vi "ODMR_MW_pulses_0.5pi(1,2,3).vi"(7 "pi/2 duration [ns]":i64=100, 9 "Measurement time [ns]":i64=100, 10 "tau/2 duration [ns]":u32, 11 "PulsePattern in":refnum<class "PulsePattern.lvclass">) -> (1 "Total duration":i64, 2 "Pulses duration":i64, 3 "PulsePattern out":refnum<class "PulsePattern.lvclass">)   [LabVIEW 2014]
uses:
  <vilib>/Swabian Instruments/Pulse Streamer/PulseStreamer/PulsePattern/PulsePattern.lvclass
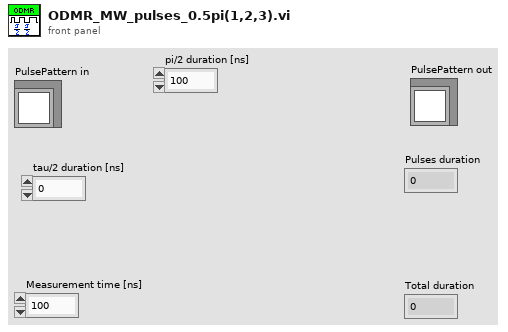
[diagram p1: front panel]
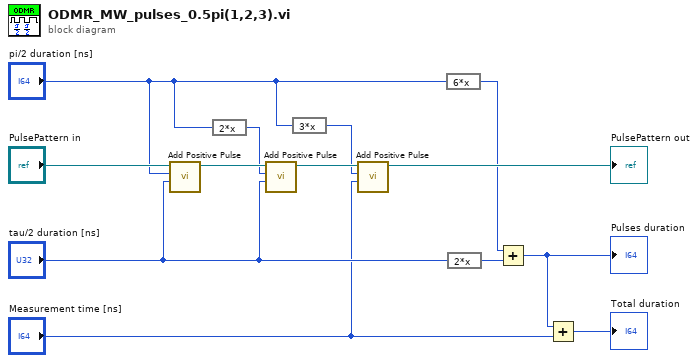
[diagram p0: block diagram]
diagram:
  n1 = call <vilib>:"Add Positive Pulse.vi"("Duration LOW"="tau/2 duration [ns]", "Duration HIGH"="pi/2 duration [ns]", "Digital Pattern in"="PulsePattern in") -> ("Digital Pattern out"=w12:refnum<class "PulsePattern.lvclass">)  [unwired: 8 in]
  n2 = expression code="2*x"("pi/2 duration [ns]") -> (w9:i64)
  n3 = call <vilib>:"Add Positive Pulse.vi"("Duration LOW"="tau/2 duration [ns]", "Duration HIGH"=w9, "Digital Pattern in"=w12) -> ("Digital Pattern out"=w11:refnum<class "PulsePattern.lvclass">)  [unwired: 8 in]
  n4 = expression code="3*x"("pi/2 duration [ns]") -> (w1:i64)
  n5 = call <vilib>:"Add Positive Pulse.vi"("Duration LOW"="Measurement time [ns]", "Duration HIGH"=w1, "Digital Pattern in"=w11) -> ("Digital Pattern out"=→"PulsePattern out":refnum<class "PulsePattern.lvclass">)  [unwired: 8 in]
  n6 = expression code="6*x"("pi/2 duration [ns]") -> (w7:i64)
  n7 = expression code="2*x"("tau/2 duration [ns]") -> (w6:u32)
  n8 = Add(x=w7, y=w6) -> (x+y=w5:i64)
  "Pulses duration" <- w5
  n9 = Add(x=w5, y="Measurement time [ns]") -> (x+y=→"Total duration":i64)
